vi "ClientSideChattingApp.vi"() -> ()   [LabVIEW 2019]
panel:
  out "error out":errorcluster
  in  "Cluster":T1
  out "Message":string
  out "Full Name":string
  out "IsSingle":bool
  out "Age":dbl
  in  "Stop from Client Side":bool
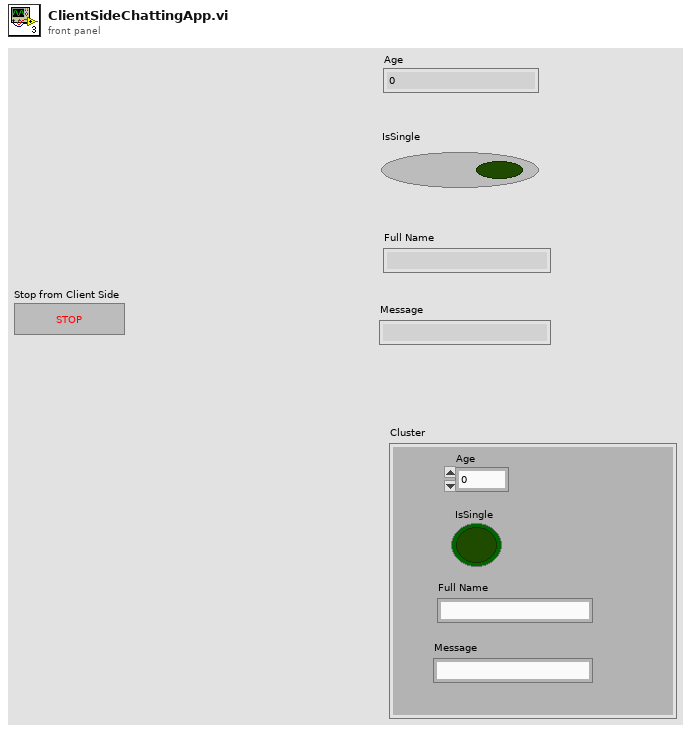
[diagram p1: front panel]
types:
  T1 = cluster{"Age":dbl, "IsSingle":bool, "Full Name":string, "Message":string}
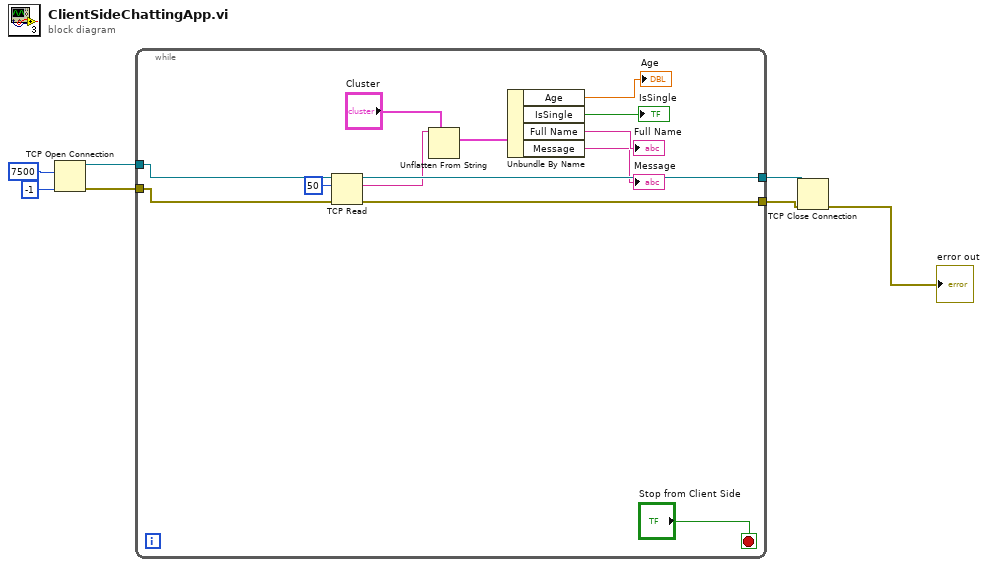
[diagram p0: block diagram]
diagram:
  n1 = TCP Open Connection(remote port or service name=u16 7500, timeout ms (60000)=-1) -> (connection ID=w5:refnum<k5>, error out=w4:errorcluster)  [unwired: 3 in]
  n2 = while {
    tunnel: w5 -> [w19]
    tunnel: w4 -> [w18]
    tunnel: [w17] -> w3
    tunnel: [w16] -> w2
    stop <- "Stop from Client Side" stop-if-true
    n3 = TCP Read(connection ID=w19, bytes to read=50, error in (no error)=w18) -> (connection ID out=w17:refnum<k5>, data out=w13:string, error out=w16:errorcluster)  [unwired: 2 in]
    n4 = Unflatten From String(type="Cluster", binary string=w13) -> (value=w12:T1)  [unwired: 3 in, 2 out]
    n5 = Unbundle By Name(w12) -> ("Age"=→"Age":dbl, "IsSingle"=→"IsSingle":bool, "Full Name"=→"Full Name":string, "Message"=→"Message":string)
  }
  n6 = TCP Close Connection(connection ID=w3, error in (no error)=w2) -> (error out=→"error out":errorcluster)  [unwired: 1 in, 1 out]
